vi "Auto Hovering with Position Prediction.vi"() -> ()   [LabVIEW 2014]
uses:
  Resources/Global.vi
panel:
  in  "Prediction?":bool=TRUE
  out "Image":T1(plugin-control)
  out "Video Loop":errorcluster
  out "Number of Particles before":i32
  out "Number of Particles after":i32
  in  "Number of Erosion":i32=30
  out "Video refresh":u32=48
  in  "ms to wait":u32
  # "Do NOT run this VI. Instead run \"AR.Drone MAIN.vi\" and select the name of this VI in the dop-down menu at the Steup tab"
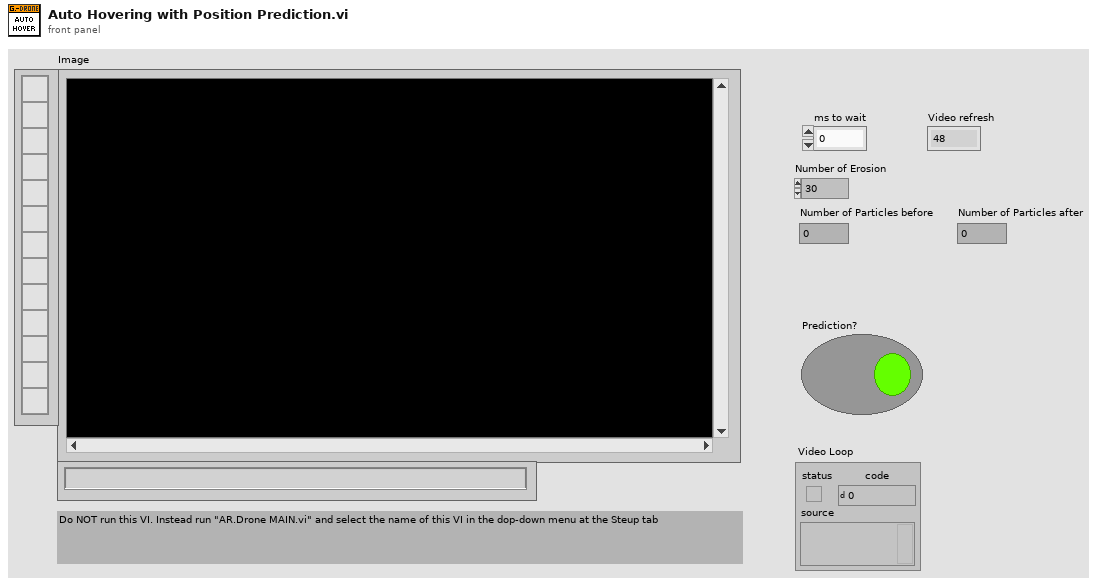
[diagram p1: front panel]
types:
  T1 = typedef "IMAQ Image.ctl" = refnum<image>
  T2 = cluster{"New Image":T1, "New Image":T1, "New Image":T1}
  T3 = cluster{"Left":dbl, "Top":dbl, "Right":dbl, "Bottom":dbl}
  T4 = cluster{"Horizontal position":dbl, "Verical position\n":dbl}
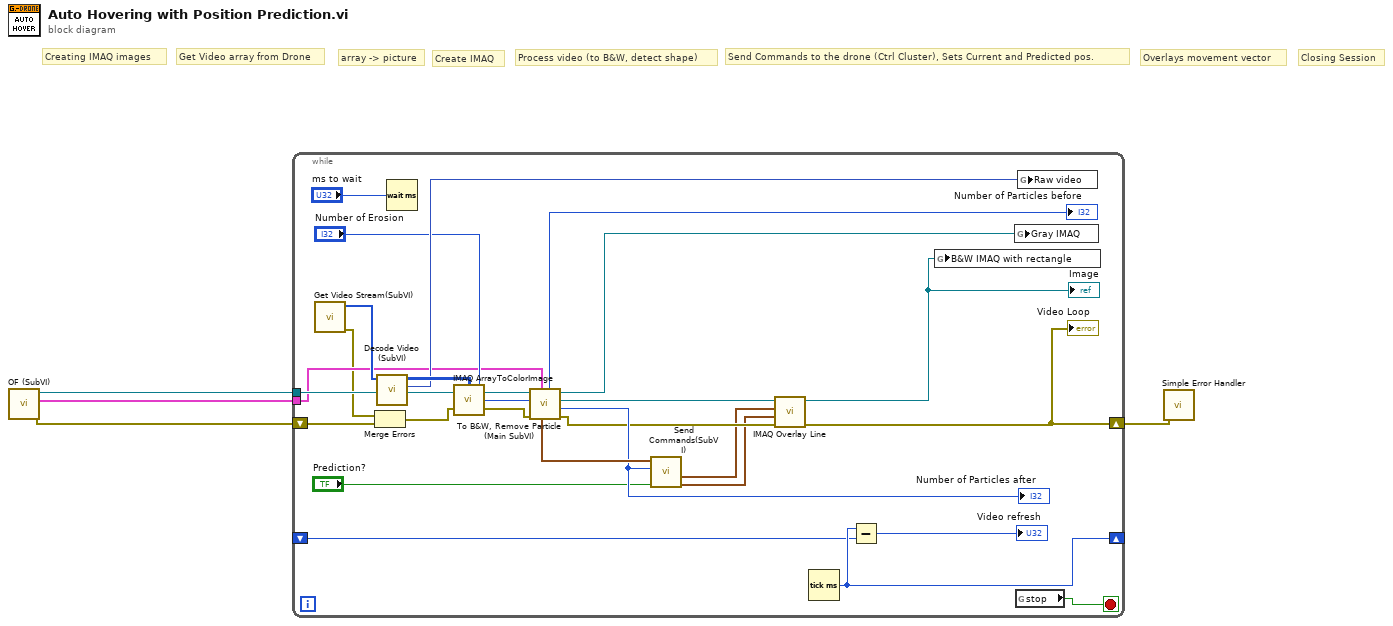
[diagram p0: block diagram]
diagram:
  # "Overlays movement vector"
  # "Send Commands to the drone (Ctrl Cluster), Sets Current and Predicted pos."
  # "Create IMAQ"
  # "Process video (to B&W, detect shape)"
  # "array -> picture"
  # "Get Video array from Drone"
  # "Closing Session"
  # "Creating IMAQ images"
  n1 = call "OF (SubVI).vi"() -> ("error out"=w2:errorcluster, "Cluster"=w3:T2, "Refnum out"=w4:T1)  [unwired: 9 in]
  n2 = while {
    shift-right: [w28] -> _
    shift-left: _ -> [w27]
    tunnel: w4 -> [w18]
    tunnel: w3 -> [w17]
    shift-right: [w9] -> w1
    shift-left: w2 -> [w8]
    stop <- w19 stop-if-true
    n3 = call "Get Video Stream(SubVI).vi"() -> ("error out"=w7:errorcluster, "ImgData"=w30:u8[])  [unwired: 10 in]
    n4 = Merge Errors(w7, w8) -> (w6:errorcluster)
    n5 = call "Decode Video (SubVI).vi"("ImgData"=w30) -> ("new picture"=w25:picture, "Array"=w29:u32[][])  [unwired: 9 in]
    n6 = Wait (ms)(milliseconds to wait="ms to wait") -> ()  [unwired: 1 out]
    n7 = call "IMAQ ArrayToColorImage"("Image Pixels (U32)"=w29, "Image"=w18, "error in (no error)"=w6) -> ("Image Out"=w24:T1, "error out"=w14:errorcluster)  [unwired: 2 in]
    n8 = call "To B&W, Remove Particle (Main SubVI).vi"("Image Reference Sources"=w17, "error in (no error)"=w14, "Number of Erosion"="Number of Erosion", "Refnum in"=w24) -> ("error out"=w12:errorcluster, "Number of Particles after"=w20:i32, "Image Out"=w13:T1, "Current Grayscale"=w16:T1, "Number of Particles before"=→"Number of Particles before":i32, "Cluster"=w22:T3)  [unwired: 1 in, 1 out]
    "Number of Particles after" <- w20
    n9 = call "Send Commands(SubVI).vi"("Prediction?"="Prediction?", "Number of Particles after"=w20, "Cluster"=w22) -> ("Predicted Position"=w11:T4, "Current position"=w10:T4)  [unwired: 7 in]
    n10 = call "IMAQ Overlay Line"("error in (no error)"=w12, "End Point"=w11, "Start Point"=w10, "Image"=w13) -> ("error out"=w9:errorcluster, "Image Out"=w5:T1)  [unwired: 6 in]
    "Video Loop" <- w9
    "Image" <- w5
    n11 = Tick Count (ms)() -> (millisecond timer value=w28:u32)
    n12 = Subtract(x=w28, y=w27) -> (x-y=→"Video refresh":u32)
    n13 = global write "Global.vi" "B&W IMAQ with rectangle"(w5) -> ()
    n14 = global write "Global.vi" "Gray IMAQ"(w16) -> ()
    n15 = global read "Global.vi" "stop"() -> (w19:bool)
    n16 = global write "Global.vi" "Raw video"(w25) -> ()
  }
  n17 = call <vilib>:"Simple Error Handler.vi"("error in (no error)"=w1) -> ()  [unwired: 4 in, 5 out]
